vi "Frame Array File Handler.vi"(8 "error in":errorcluster, 10 "selected frame array file":path, 11 "configuration file page data":T1 {"custom device ref" format="%.0x"}) -> (0 "error out":errorcluster, 3 "configuration file page data out":T1 {"custom device ref" format="%.0x"})   [LabVIEW 2020, in "AIM ARINC 664 System Explorer.lvlib" / "Implementation.lvlib"]
uses:
  Implementation.lvlib
  Types/Configuration File Page Data.ctl
  Types/Path Control.ctl
  Types/Browse Button.ctl
  <vilib>/NI VeriStand/Custom Device API/Custom Device Item Ref.ctl
  Scripting/AIM ARINC 664 Scripting.lvlib
  Import/AIM ARINC 664 Import.lvlib
  <vilib>/NI VeriStand/Custom Device API/Custom Device API.lvlib
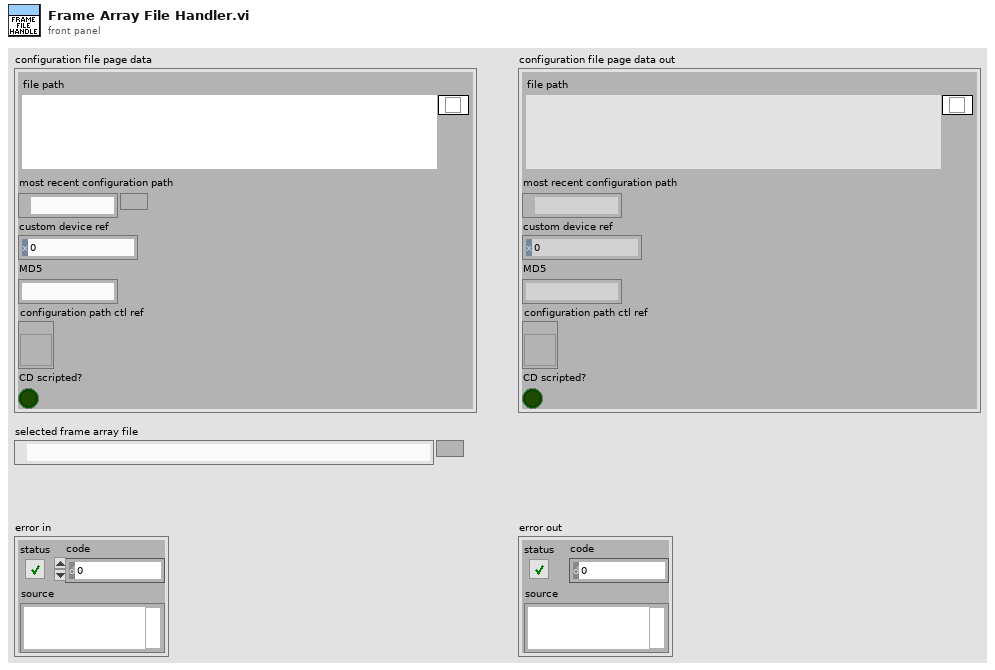
[diagram p1: front panel]
types:
  T1 = typedef "AIM ARINC 664 System Explorer.lvlib/Implementation.lvlib/Configuration File Page Data.ctl" = cluster{"Parameters":T2, "most recent configuration path":path, "custom device ref":T4, "MD5":string, "configuration path ctl ref":refnum<vi>, "CD scripted?":bool}
  T2 = typedef "AIM ARINC 664 System Explorer.lvlib/Implementation.lvlib/Path Control.ctl" = cluster{"file path":path, "Browse":T3}
  T3 = typedef "AIM ARINC 664 System Explorer.lvlib/Implementation.lvlib/Browse Button.ctl" = bool
  T4 = typedef "Custom Device API.lvlib/Custom Device Item Ref.ctl" = u64
  T5 = typedef "Port Session Configuration.ctl" = cluster{"boardId":u32, "session_tx_generic":T6[], "session_rx_monitor":T7[]}
  T6 = typedef "session_tx_generic.ctl" = cluster{"portId":u32, "QueueSizeIn":u32}
  T7 = typedef "session_rx_monitor.ctl" = cluster{"portId":u32, "DefaultCronoMode":u32, "GlbMonBufferSizeIn":u32, "CaptureMode":u32, "MaxFileSize MB (1)":u32, "Strobe":u32, "TriggerPosition":u32}
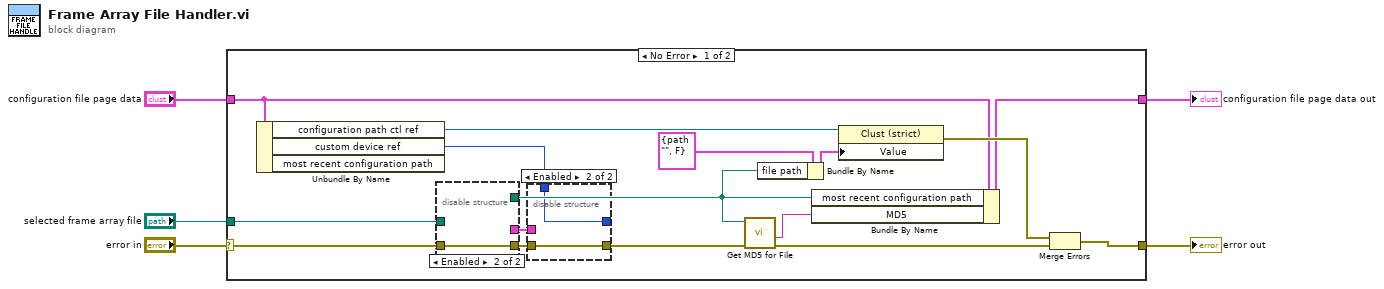
[diagram p0: block diagram]
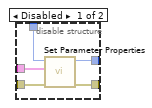
[diagram p2: hidden frame]
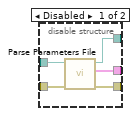
[diagram p3: hidden frame]
diagram:
  n1 = case shown="No Error" "error in" {
    selector: "error in" -> [w19 w35]
    tunnel: "configuration file page data" -> [w18 w36]
    tunnel: "selected frame array file" -> [w20 _]
    tunnel: [w17 w36] -> w2
    tunnel: [w12 w35] -> w1
    frame No Error {
      n2 = Unbundle By Name(w18) -> ("configuration path ctl ref"=w7:refnum<vi>, "custom device ref"=w9:T4)  [unwired: 1 out]
      n3 = disable-structure shown="Enabled" {
        disable-tunnel: w20 -> [w33 _]
        disable-tunnel: w19 -> [w32 w34]
        disable-tunnel: [w31 _] -> w16
        disable-tunnel: [w30 _] -> w11
        disable-tunnel: [w29 w34] -> w8
        frame Disabled {
          n4 = call "Parse Parameters File.vi"("error in"=w32, "path to XML document"=w33) -> ("error out"=w29:errorcluster, "port sessions"=w31:T5, "path to XML document out"=w30:path)  [unwired: 7 in]
        }
        frame Enabled {
        }
      }
      n5 = disable-structure shown="Enabled" {
        disable-tunnel: w16 -> [w26 _]
        disable-tunnel: [w25 w27] -> w6
        disable-tunnel: w9 -> [w24 w28]
        disable-tunnel: w8 -> [w23 w27]
        disable-tunnel: [w22 w28] -> _
        frame Disabled {
          n6 = call "Set Parameter Properties.vi"("custom device ref in"=w24, "port sessions"=w26, "error in"=w23) -> ("custom device ref out"=w22:T4, "error out"=w25:errorcluster)  [unwired: 6 in]
        }
        frame Enabled {
        }
      }
      n7 = call "Get MD5 for File.vi"("error in"=w6, "Path"=w11) -> ("error out"=w10:errorcluster, "MD5"=w15:string)  [unwired: 8 in]
      n8 = Bundle By Name(cluster=T2 {"file path"=path "", "Browse"=FALSE} ("Path"), "file path"=w11) -> (w13:T2)
      n9 = Bundle By Name(cluster=w18, "most recent configuration path"=w11, "MD5"=w15) -> (w17:T1)
      n10 = property class="Clust (strict)"(reference=w7, "Value"=w13) -> (error out=w21:errorcluster)  [unwired: 1 in, 1 out]
      n11 = Merge Errors(w21, w10) -> (w12:errorcluster)
    }
    frame Error {
    }
  }
  "configuration file page data out" <- w2
  "error out" <- w1
